vi "Query Client Errors.vi"(8 "error in":errorcluster, 11 "NATS Client":refnum<class "NATS Client.lvclass">) -> (0 "error out":errorcluster, 3 "errors":errorcluster[](array[cluster]))   [LabVIEW 2024, in "NATS Client.lvlib" / "NATS Client.lvclass"]
doc: "Return Client asynchronous daemon errors."
uses:
  NATS Client.lvclass
  NATS Client.lvclass/NATS Client.ctl
  Get error queue.vi
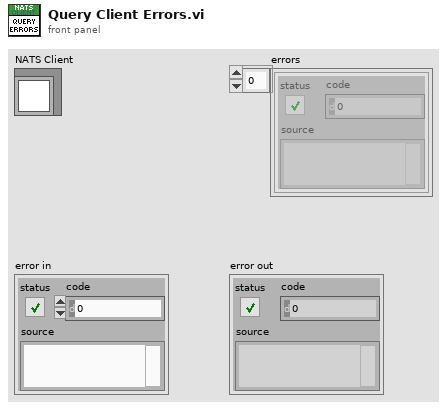
[diagram p1: front panel]
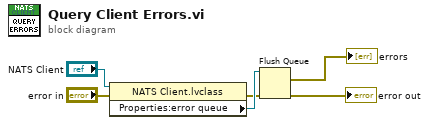
[diagram p0: block diagram]
diagram:
  n1 = property class="NATS Client.lvclass"(reference="NATS Client", error in="error in") -> (error out=w4:errorcluster, "Properties:error queue"=w5:refnum<queue>)  [unwired: 1 out]
  n2 = Flush Queue(queue=w5, error in (no error)=w4) -> (remaining elements=→"errors":errorcluster[], error out=→"error out":errorcluster)  [unwired: 1 out]
